vi "Get TCP Messaging API.vi"(8 "error in (no error)":errorcluster, 11 "Vecto in":refnum<class "Vecto.lvclass">) -> (0 "error out":errorcluster, 2 "TCP Messaging API":refnum<class "TCPMessageAPI.lvclass">, 3 "Vecto out":refnum<class "Vecto.lvclass">)   [LabVIEW 2020, in "Vecto.lvlib" / "Vecto.lvclass"]
uses:
  Vecto.lvclass
  TCPMessageService/TCPMessageAPI.lvclass
  Vecto.lvclass/Vecto.ctl
  TCPMessaging/TCPMessaging.lvclass
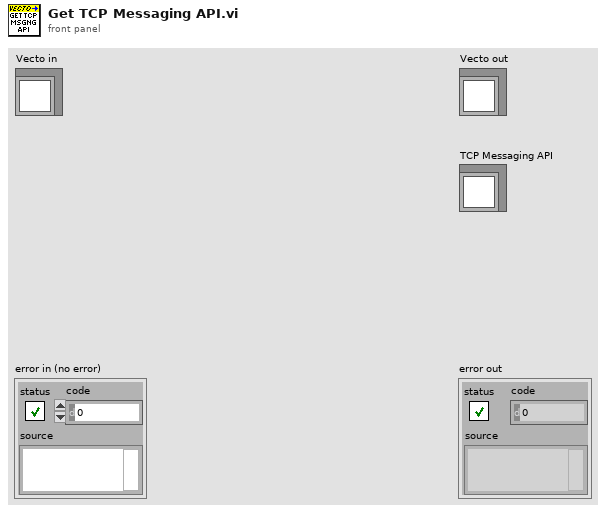
[diagram p1: front panel]
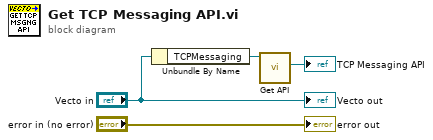
[diagram p0: block diagram]
diagram:
  n1 = Unbundle By Name("Vecto in") -> ("TCPMessaging"=w2:refnum<class "TCPMessaging.lvclass">)
  n2 = call "Get API.vi"("TCPMessaging in"=w2) -> ("TCP Messaging API"=→"TCP Messaging API":refnum<class "TCPMessageAPI.lvclass">)  [unwired: 8 in, 2 out]
  "error out" <- "error in (no error)"
  "Vecto out" <- "Vecto in"
